vi "Climb Teleop Handler.vi"() -> ()   [LabVIEW 2023]
uses:
  Teleop Util/Climb States.ctl
  19f54aaa-fd46-4467-b46d-a9580f8c6a79.vi
  196f44d3-2ce2-4218-9bff-502957a5b400.vi
  <vilib>/Rock Robotics/WPI/Utilities/WPI_GetSetVariantRefNum.vi
panel:
  out "s? t:f":T1
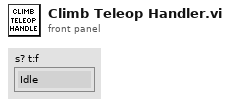
[diagram p1: front panel]
types:
  T1 = typedef "Climb States.ctl" = enum16{"Idle", "Deploy", "Undeploy", "Manual Overrides"}
  T2 = typedef "WPI_JoystickDevRef.ctl" = cluster{"Device":T3}
  T3 = typedef "WPI_JoystickDeviceEnum.ctl" = enum16{"USB 0", "USB 1", "USB 2", "USB 3", "USB 4", "USB 5"}
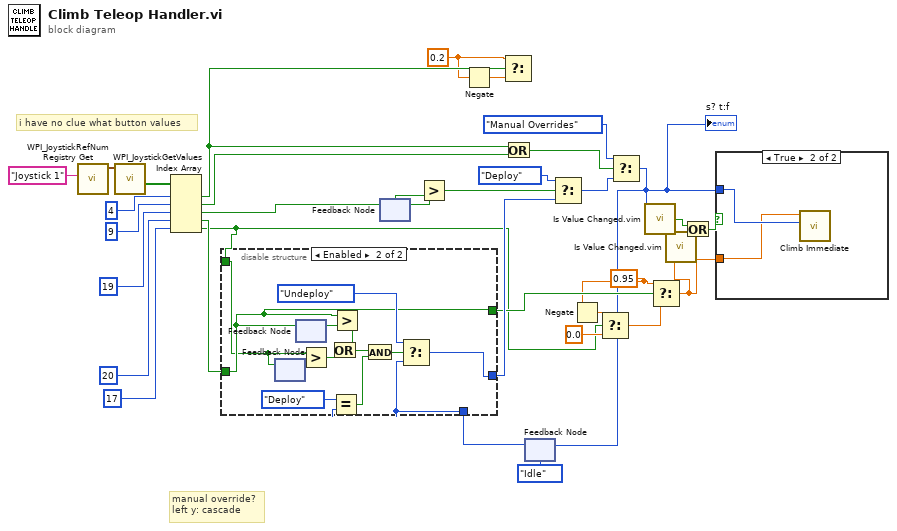
[diagram p0: block diagram]
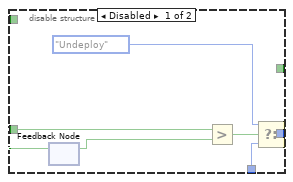
[diagram p2: hidden frame]
diagram:
  w4 = 0.95 ("t")
  w14 = 0.2 ("t")
  # "manual override?\nleft y: cascade"
  # "i have no clue what button values"
  n1 = call <vilib>:"WPI_JoystickRefNum Registry Get.vi"("refnum name"="Joystick 1") -> ("JoystickDevRef"=w33:T2)  [unwired: 1 in, 9 out]
  n2 = call <vilib>:"WPI_JoystickGetValues.vi"("JoystickDevRef"=w33) -> ("Buttons"=w32:bool[])  [unwired: 6 in, 4 out]
  n3 = Index Array(array=w32, index #1=4 ("index"), index #2=9 ("index"), index #3=19 ("index"), index #4=20 ("index"), index #5=17 ("index")) -> (element #1=w15:bool, element #2=w16:bool, element #3=w30:bool, element #4=w26:bool, element #5=w1:bool)
  n4 = feedback-in #1(w30) -> ()
  n5 = feedback #1() -> (w29:bool)  [unwired: 1 in]
  n6 = Greater?(x=w30, y=w29) -> (0:w31:bool)
  n7 = Negate(x=w14) -> (-x=w13:dbl)
  n8 = Select(t=w14, s=w15, f=w13) -> ()  [unwired: 1 out]
  n9 = Or(x=w15, y=w16) -> (x .or. y?=w17:bool)
  n10 = feedback #2(Climb_States."Idle") -> (w24:T1)
  n11 = disable-structure shown="Enabled" {
    disable-tunnel: [w40 w47] -> w27
    disable-tunnel: w26 -> [w39 w46]
    disable-tunnel: w24 -> [w35 w48]
    disable-tunnel: [_ w46] -> w8
    disable-tunnel: w1 -> [_ w41]
    frame Disabled {
      n12 = feedback #3() -> (w38:bool)  [unwired: 1 in]
      n13 = feedback-in #3(w39) -> ()
      n14 = Greater?(x=w39, y=w38) -> (0:w37:bool)
      n15 = Select(t=Climb_States."Undeploy", s=w37, f=w35) -> (s? t:f=w40:T1)
    }
    frame Enabled {
      n16 = feedback #4() -> (w43:bool)  [unwired: 1 in]
      n17 = feedback-in #4(w41) -> ()
      n18 = feedback #5() -> (w51:bool)  [unwired: 1 in]
      n19 = feedback-in #5(w46) -> ()
      n20 = Greater?(x=w41, y=w43) -> (0:w42:bool)
      n21 = Equal?(x=Climb_States."Deploy", y=w48) -> (x = y?=w52:bool)
      n22 = Greater?(x=w46, y=w51) -> (0:w44:bool)
      n23 = Or(x=w44, y=w42) -> (x .or. y?=w45:bool)
      n24 = And(x=w45, y=w52) -> (x .and. y?=w50:bool)
      n25 = Select(t=Climb_States."Undeploy", s=w50, f=w48) -> (s? t:f=w47:T1)
    }
  }
  n26 = Select(t=Climb_States."Deploy", s=w31, f=w27) -> (s? t:f=w23:T1)
  n27 = Negate(x=w4) -> (-x=w3:dbl)
  n28 = Select(t=w3, s=w1, f=0.0) -> (s? t:f=w5:dbl)
  n29 = Select(t=Climb_States."Manual Overrides", s=w17, f=w23) -> (s? t:f=w7:T1)
  "s? t:f" <- w7
  n30 = feedback-in #2(w7) -> ()
  n31 = call "Is Value Changed.vim"("value"=w7) -> ("changed or first call?"=w11:bool)
  n32 = Select(t=w4, s=w8, f=w5) -> (s? t:f=w10:dbl)
  n33 = call "Is Value Changed.vim"("value"=w10) -> ("changed or first call?"=w9:bool)
  n34 = Or(x=w11, y=w9) -> (x .or. y?=w12:bool)
  n35 = case shown="True" w12 {
    tunnel: w7 -> [_ w55]
    tunnel: w10 -> [_ w54]
    frame False {
    }
    frame True {
      n36 = call "Climb Immediate.vi"("Climb States"=w55, "Setpoint"=w54) -> ()  [unwired: 9 in, 1 out]
    }
  }
